vi "GET_Show.vi"(8 "error in (no error)":errorcluster {"code" min=0 max=0}, 11 "Settings.lvclass in":refnum<class "Settings.lvclass">) -> (0 "error out":errorcluster {"code" min=0 max=0}, 1 "Show Terminals?":bool, 2 "Show LayerTab?":bool, 3 "Settings.lvclass out":refnum<class "Settings.lvclass">)   [LabVIEW 2021, in "Settings.lvclass"]
uses:
  <resource>/plugins/NIIconEditor/Class/Settings/Settings.lvclass
  <resource>/plugins/NIIconEditor/Class/Settings/Settings.lvclass/Settings.ctl
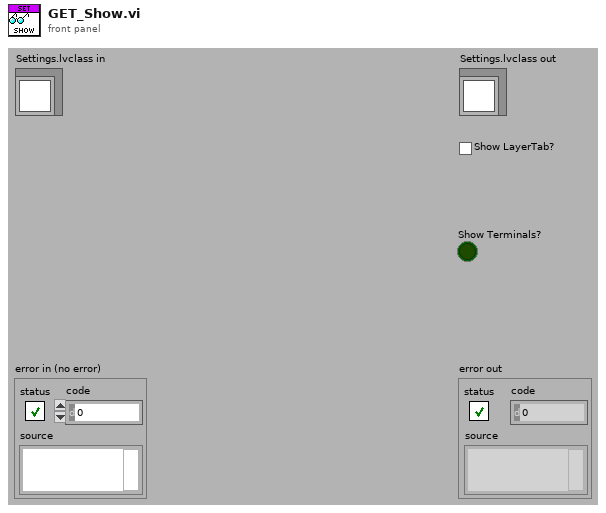
[diagram p1: front panel]
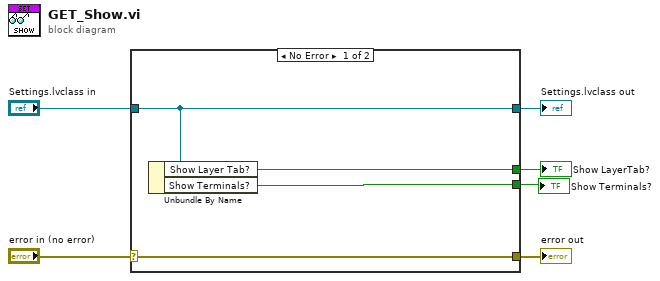
[diagram p0: block diagram]
diagram:
  n1 = case shown="No Error" "error in (no error)" {
    selector: "error in (no error)" -> [w10 w11]
    tunnel: [w10 w11] -> w5
    tunnel: [w9 w12] -> w3
    tunnel: "Settings.lvclass in" -> [w9 w12]
    tunnel: [w8 _] -> w2
    tunnel: [w7 _] -> w1
    frame No Error {
      n2 = Unbundle By Name(w9) -> ("Show Layer Tab?"=w8:bool, "Show Terminals?"=w7:bool)
    }
    frame Error {
    }
  }
  "error out" <- w5
  "Settings.lvclass out" <- w3
  "Show LayerTab?" <- w2
  "Show Terminals?" <- w1
